vi "Configure Frequency.vi"(5 "Sweep time (ms)":dbl=10.0 caption="Sweep time for zero span (ms)", 7 "Mode (Center/Span)":enum16{"Center/Span", "Start/Stop"}(ring), 8 "error in (no error)":errorcluster, 9 "Span/Stop Frequency [Hz]":dbl, 10 "Center/Start Frequency [Hz]":dbl, 11 "SA-ESA in":refnum<class "SA-ESA.lvclass">) -> (0 "error out":errorcluster, 3 "SA-ESA out":refnum<class "SA-ESA.lvclass">)   [LabVIEW 2020, in "SA-ESA.lvclass"]
uses:
  SA-ESA.lvclass
  C:/Sandbox/RF Bench/Source Code/WiSpry Test Framework/Instruments/Spectrum Analyzer/Spectrum Analyzer.lvclass
  C:/Sandbox/RF Bench/Source Code/WiSpry Test Framework/Instruments/Instrument.lvclass
  Spectrum Analyzer.lvclass/Spectrum Analyzer.ctl
  Instrument.lvclass/Instrument.ctl
  Spectrum Analyzer.lvclass
  Instrument.lvclass
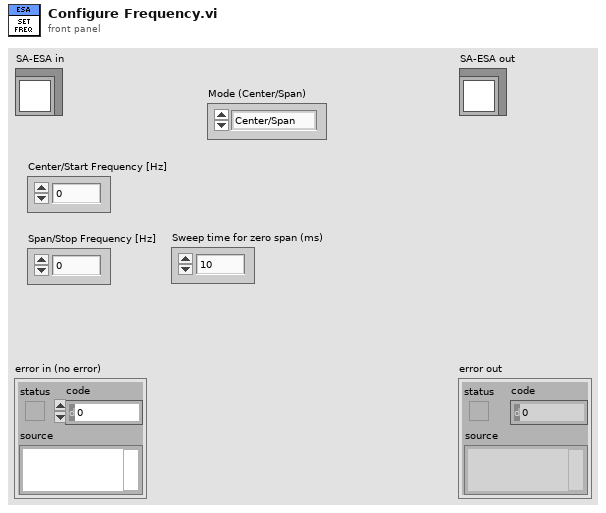
[diagram p1: front panel]
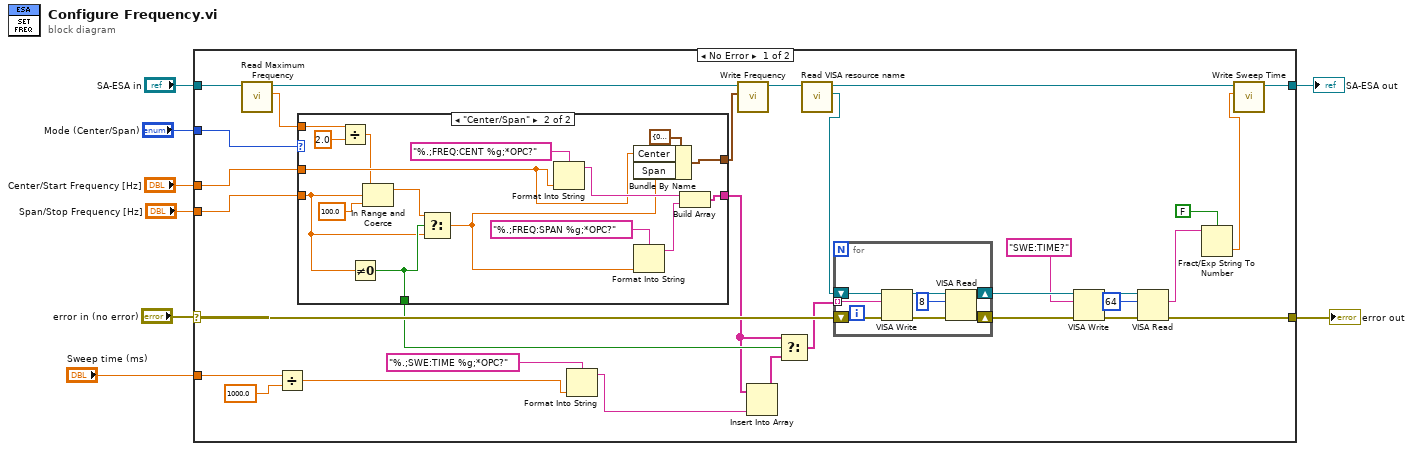
[diagram p0: block diagram]
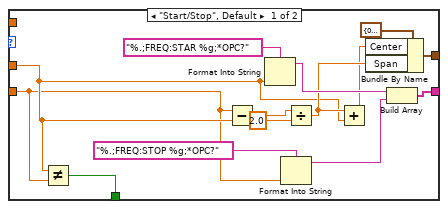
[diagram p2: hidden frame]
diagram:
  n1 = case shown="No Error" "error in (no error)" {
    selector: "error in (no error)" -> [w33 w78]
    tunnel: "Mode (Center/Span)" -> [w39 _]
    tunnel: "Center/Start Frequency [Hz]" -> [w38 _]
    tunnel: "Span/Stop Frequency [Hz]" -> [w37 _]
    tunnel: "SA-ESA in" -> [w20 w79]
    tunnel: [w22 w79] -> w3
    tunnel: [w21 w78] -> w2
    tunnel: "Sweep time (ms)" -> [w17 _]
    frame No Error {
      n2 = call "Read Maximum Frequency.vi"("Spectrum Analyzer in"=w20) -> ("Maximum Frequency"=w18:dbl, "Spectrum Analyzer out"=w19:refnum<class "SA-ESA.lvclass">)  [unwired: 9 in]
      n3 = Divide(x=w17, y=1000.0) -> (x/y=w13:dbl)
      n4 = case shown="\"Center/Span\"" w39 {
        tunnel: w38 -> [w50 w73]
        tunnel: w37 -> [w49 w64]
        tunnel: [w53 w72] -> w10
        tunnel: [w54 w74] -> w36
        tunnel: w18 -> [_ w68]
        tunnel: [w48 w65] -> w15
        frame "Start/Stop", Default {
          n5 = Not Equal?(x=w50, y=w49) -> (x != y?=w48:bool)
          n6 = Subtract(x=w49, y=w50) -> (x-y=w58:dbl)
          n7 = Format Into String(format string="%.;FREQ:STAR %g;*OPC?", w50) -> (resulting string=w60:string)  [unwired: 2 in, 1 out]
          n8 = Format Into String(format string="%.;FREQ:STOP %g;*OPC?", w49) -> (resulting string=w52:string)  [unwired: 2 in, 1 out]
          n9 = Divide(x=w58, y=2.0) -> (x/y=w56:dbl)
          n10 = Add(x=w56, y=w50) -> (x+y=w55:dbl)
          n11 = Bundle By Name(cluster=cluster{"Center":dbl, "Span":dbl} {"Center"=0.0, "Span"=0.0} ("Frequency"), "Center"=w55, "Span"=w56) -> (w54:cluster{"Center":dbl, "Span":dbl})
          n12 = Build Array(w60, w52) -> (w53:string[])
        }
        frame "Center/Span" {
          n13 = Divide(x=w68, y=2.0) -> (x/y=w66:dbl)
          n14 = Not Equal To 0?(x=w64) -> (x != 0?=w65:bool)
          n15 = In Range and Coerce(upper limit=w66, x=w64, lower limit=100.0) -> (coerced(x)=w63:dbl)  [unwired: 1 out]
          n16 = Select(t=w63, s=w65, f=w64) -> (s? t:f=w62:dbl)
          n17 = Format Into String(format string="%.;FREQ:CENT %g;*OPC?", w73) -> (resulting string=w76:string)  [unwired: 2 in, 1 out]
          n18 = Bundle By Name(cluster=cluster{"Center":dbl, "Span":dbl} {"Center"=0.0, "Span"=0.0} ("Frequency"), "Center"=w73, "Span"=w62) -> (w74:cluster{"Center":dbl, "Span":dbl})
          n19 = Format Into String(format string="%.;FREQ:SPAN %g;*OPC?", w62) -> (resulting string=w70:string)  [unwired: 2 in, 1 out]
          n20 = Build Array(w76, w70) -> (w72:string[])
        }
      }
      n21 = Format Into String(format string="%.;SWE:TIME %g;*OPC?", w13) -> (resulting string=w12:string)  [unwired: 2 in, 1 out]
      n22 = call "Write Frequency.vi"("Frequency"=w36, "Spectrum Analyzer in"=w19) -> ("Spectrum Analyzer out"=w35:refnum<class "SA-ESA.lvclass">)  [unwired: 9 in]
      n23 = Insert Into Array(array=w10, new element=w12) -> (w11:string[])  [unwired: 1 in]
      n24 = Select(t=w10, s=w15, f=w11) -> (s? t:f=w9:string[])
      n25 = call "Read VISA resource name.vi"("Instrument in"=w35) -> ("VISA resource name"=w34:refnum<visa-resource-name>, "Instrument out"=w24:refnum<class "SA-ESA.lvclass">)  [unwired: 9 in]
      n26 = for {
        tunnel: w9 -> [w40] mode=indexing
        shift-right: [w41] -> w31
        shift-left: w34 -> [w47]
        shift-right: [w42] -> w32
        shift-left: w33 -> [w46]
        n27 = VISA Write(VISA resource name=w47, write buffer=w40, error in (no error)=w46) -> (VISA resource name out=w44:refnum<visa-resource-name>, error out=w45:errorcluster)  [unwired: 1 out]
        n28 = VISA Read(VISA resource name=w44, byte count=u32 8, error in (no error)=w45) -> (VISA resource name out=w41:refnum<visa-resource-name>, error out=w42:errorcluster)  [unwired: 2 out]
      }
      n29 = VISA Write(VISA resource name=w31, write buffer="SWE:TIME?", error in (no error)=w32) -> (VISA resource name out=w28:refnum<visa-resource-name>, error out=w29:errorcluster)  [unwired: 1 out]
      n30 = VISA Read(VISA resource name=w28, byte count=u32 64, error in (no error)=w29) -> (read buffer=w25:string, error out=w21:errorcluster)  [unwired: 2 out]
      n31 = Fract/Exp String To Number(use system decimal point (T)=FALSE, string=w25) -> (number=w23:dbl)  [unwired: 2 in, 1 out]
      n32 = call "Write Sweep Time.vi"("Sweep Time"=w23, "Spectrum Analyzer in"=w24) -> ("Spectrum Analyzer out"=w22:refnum<class "SA-ESA.lvclass">)  [unwired: 9 in]
    }
    frame Error {
    }
  }
  "error out" <- w2
  "SA-ESA out" <- w3
